vi "Close.vi"(8 "error in (no error)":errorcluster, 11 "Data in":refnum<class "SharedVariable_Bus.lvclass">) -> (0 "error out":errorcluster, 3 "Data out":refnum<class "SharedVariable_Bus.lvclass">)   [LabVIEW 2021, in "SharedVariable_Bus.lvclass"]
doc: "Abstract Data Classes 2.1.1.12\nTim Streeter - TSA\nCopyright (c) 2024, TSA"
uses:
  SharedVariable_Bus.lvclass
  C:/Program Files (x86)/National Instruments/LabVIEW 2021/vi.lib/TSA/Omni-Bus/Omni-Bus/Bus Access/Bus_Access.lvclass
  <vilib>/TSA/Omni-Bus/Omni-Bus/Bus Access/Bus_Access.lvclass/Bus_Access.ctl
  <vilib>/TSA/Omni-Bus/Omni-Bus/Bus Access/Properties/Read Values.vi
  <vilib>/TSA/Abstract Data Classes/Abs_Types/Type/Abs_Type.lvclass
  SharedVariable_Bus.lvclass/SharedVariable_Bus.ctl
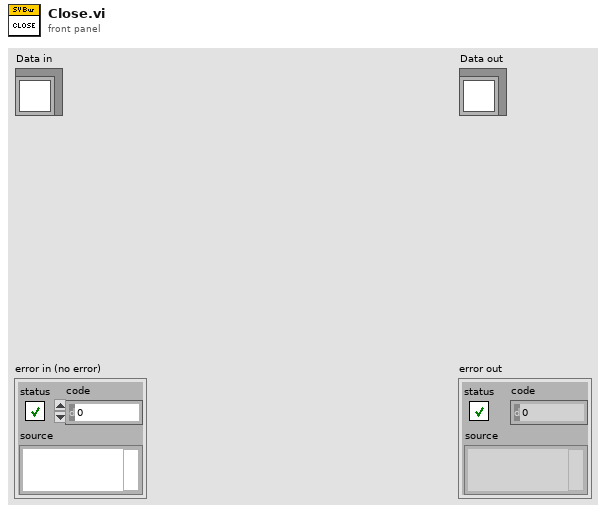
[diagram p1: front panel]
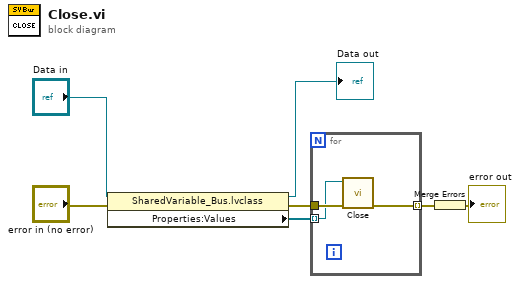
[diagram p0: block diagram]
diagram:
  n1 = property class="SharedVariable_Bus.lvclass"(reference="Data in", error in="error in (no error)") -> (reference out=→"Data out":refnum<class "SharedVariable_Bus.lvclass">, error out=w4:errorcluster, "Properties:Values"=w5:refnum<class "Abs_Type.lvclass">[])
  n2 = for {
    tunnel: w5 -> [w9] mode=indexing
    tunnel: w4 -> [w10]
    tunnel: [w8] -> w3 mode=indexing
    n3 = call-dynamic "Close.vi"("error in (no error)"=w10, "Data in"=w9) -> ("error out"=w8:errorcluster)  [unwired: 8 in, 1 out]
  }
  n4 = Merge Errors(w3) -> (→"error out":errorcluster)
